vi "eval_simple_formula.vi"() -> ()   [LabVIEW 2021]
uses:
  state_def.ctl
panel:
  out "error out":errorcluster
  in  "formula":string="123"
  out "result":dbl
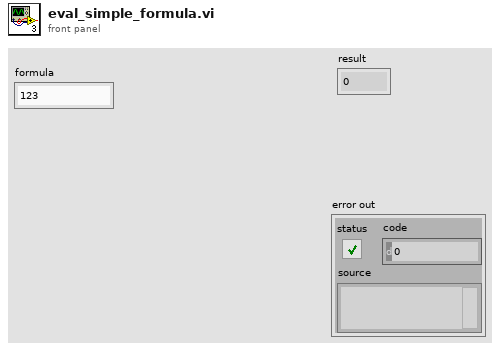
[diagram p1: front panel]
types:
  T1 = typedef "state_def.ctl" = enum16{"Init", "Construct Number", "Check Stack Priority 1", "Check Stack Priority 2", "Push", "Calculate"}
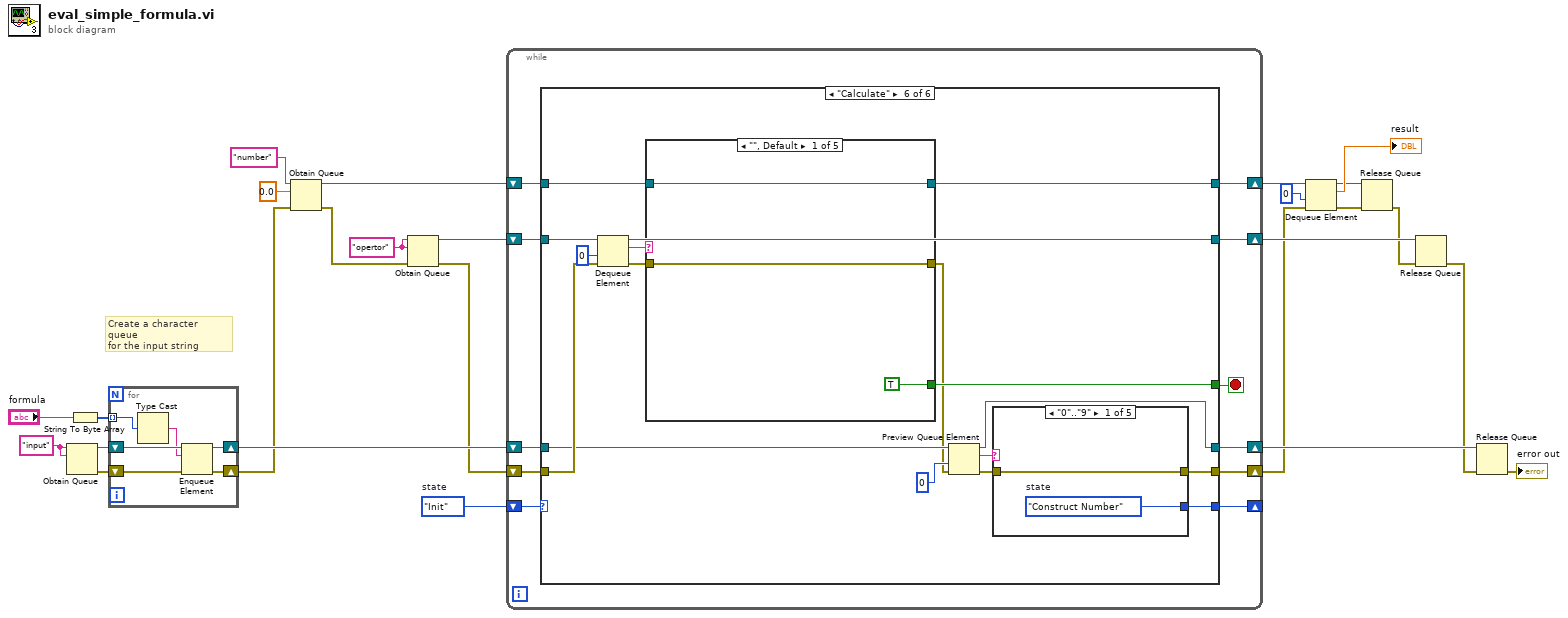
[diagram p0: block diagram]
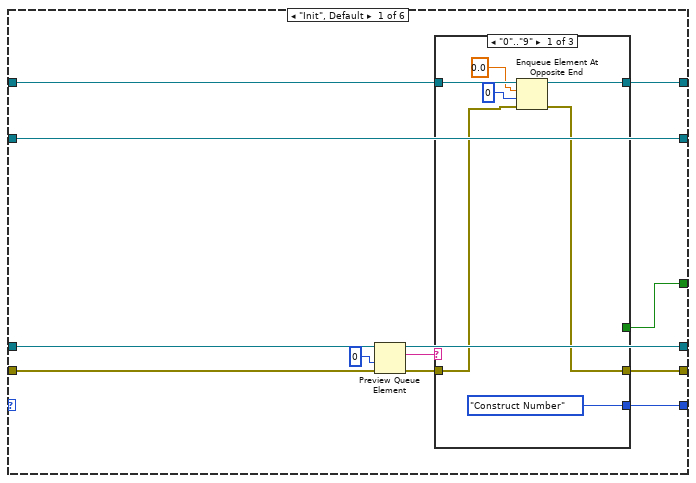
[diagram p2: hidden frame]
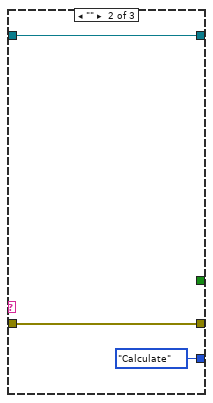
[diagram p3: hidden frame]
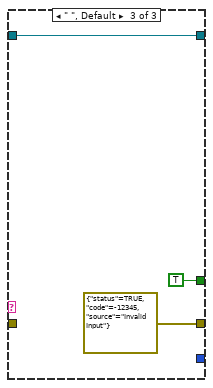
[diagram p4: hidden frame]
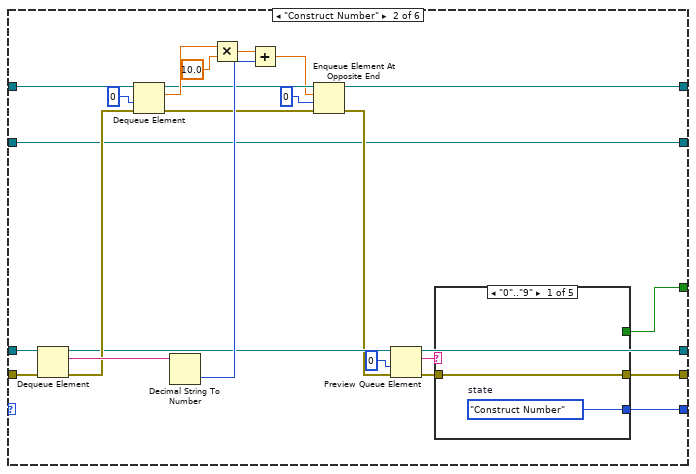
[diagram p5: hidden frame]
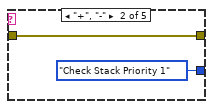
[diagram p6: hidden frame]
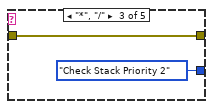
[diagram p7: hidden frame]
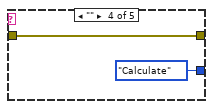
[diagram p8: hidden frame]
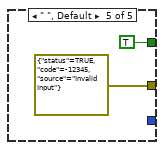
[diagram p9: hidden frame]
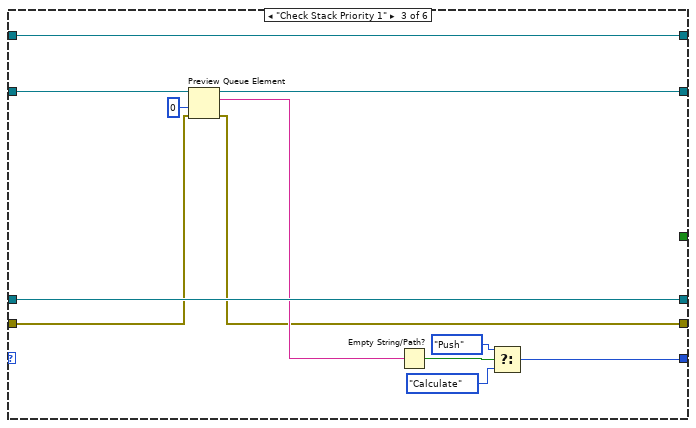
[diagram p10: hidden frame]
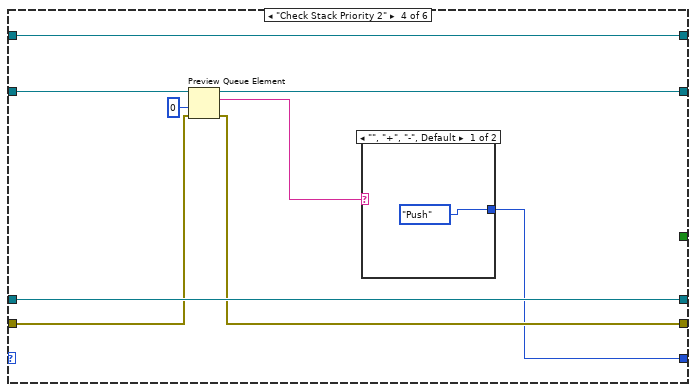
[diagram p11: hidden frame]
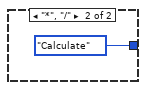
[diagram p12: hidden frame]
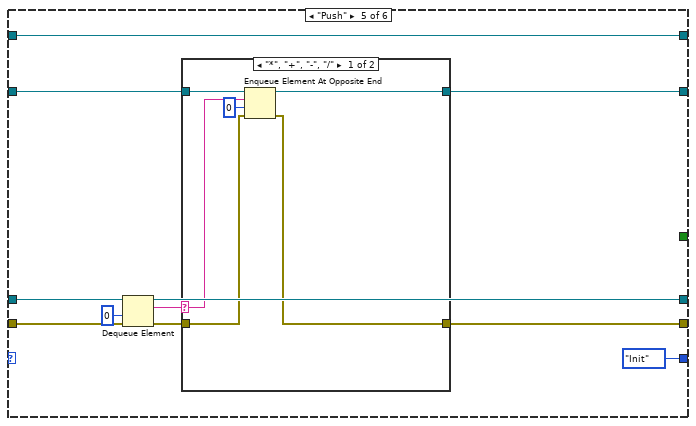
[diagram p13: hidden frame]
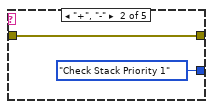
[diagram p15: hidden frame]
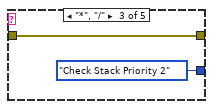
[diagram p16: hidden frame]
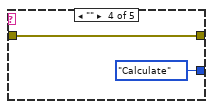
[diagram p17: hidden frame]
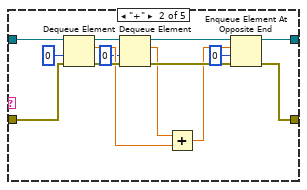
[diagram p19: hidden frame]
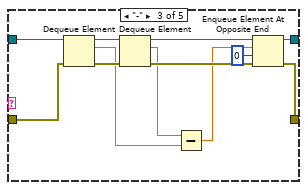
[diagram p20: hidden frame]
diagram:
  w18 = "input" ("name (unnamed)")
  w21 = "opertor" ("name (unnamed)")
  w2 = state_def."Init"  # state
  # "Create a character queue \nfor the input string"
  n1 = Obtain Queue(name (unnamed)=w18, element data type=w18) -> (queue out=w17:refnum<queue>, error out=w14:errorcluster)  [unwired: 3 in, 1 out]
  n2 = String To Byte Array(string="formula") -> (unsigned byte array=w25:u8[])
  n3 = for {
    tunnel: w25 -> [w32] mode=indexing
    shift-right: [w29] -> w16
    shift-left: w17 -> [w31]
    shift-right: [w27] -> w13
    shift-left: w14 -> [w28]
    n4 = Type Cast(x=w32) -> (*(type *) &x=w30:string)  [unwired: 1 in]
    n5 = Enqueue Element(queue=w31, element=w30, error in (no error)=w28) -> (queue out=w29:refnum<queue>, error out=w27:errorcluster)  [unwired: 1 in, 1 out]
  }
  n6 = Obtain Queue(name (unnamed)="number", element data type=0.0 ("current number"), error in (no error)=w13) -> (queue out=w22:refnum<queue>, error out=w12:errorcluster)  [unwired: 2 in, 1 out]
  n7 = Obtain Queue(name (unnamed)=w21, element data type=w21, error in (no error)=w12) -> (queue out=w20:refnum<queue>, error out=w11:errorcluster)  [unwired: 2 in, 1 out]
  n8 = while {
    shift-right: [w42] -> w8
    shift-left: w22 -> [w43]
    shift-right: [w40] -> w19
    shift-left: w20 -> [w39]
    shift-right: [w35] -> _
    shift-left: w2 -> [w33]
    shift-right: [w34] -> w15
    shift-left: w16 -> [w38]
    shift-right: [w37] -> w5
    shift-left: w11 -> [w41]
    stop <- w36 stop-if-true
    n9 = case shown="\"Calculate\"" w33 {
      tunnel: w43 -> [w55 w91 w115 w124 w137 w162]
      tunnel: [w54 w82 w115 w124 w137 w160] -> w42
      tunnel: w41 -> [w49 w81 w106 w119 w135 w157]
      tunnel: [w45 w69 w111 w120 w131 w158] -> w40
      tunnel: w39 -> [w45 w69 w113 w122 w132 w161]
      tunnel: [w53 w74 w105 w118 w130 w147] -> w37
      tunnel: [w44 w76 w114 w123 w134 w146] -> w34
      tunnel: w38 -> [w52 w93 w114 w123 w136 w150]
      tunnel: [w50 w70 _ _ _ w155] -> w36
      tunnel: [w46 w75 w108 w116 state_def."Init" ("f") w148] -> w35
      frame "Init", Default {
        n10 = Preview Queue Element(queue=w52, timeout in ms (-1)=0, error in (no error)=w49) -> (queue out=w44:refnum<queue>, element=w47:string, error out=w48:errorcluster)  [unwired: 1 out]
        n11 = case shown="\"0\"..\"9\"" w47 {
          tunnel: w55 -> [w62 w64 w66]
          tunnel: [w60 w64 w66] -> w54
          tunnel: w48 -> [w59 w65 _]
          tunnel: [w58 w65 errorcluster {"status"=TRUE, "code"=-12345, "source"="Invalid Input"} ("error out")] -> w53
          tunnel: [_ _ TRUE] -> w50
          tunnel: [state_def."Construct Number" ("state") state_def."Calculate" ("state") _] -> w46
          frame "0".."9" {
            n12 = Enqueue Element At Opposite End(queue=w62, element=0.0, timeout in ms (-1)=0, error in (no error)=w59) -> (queue out=w60:refnum<queue>, error out=w58:errorcluster)  [unwired: 1 out]
          }
          frame "" {
          }
          frame " ", Default {
          }
        }
      }
      frame "Construct Number" {
        n13 = Dequeue Element(queue=w93, error in (no error)=w81) -> (queue out=w78:refnum<queue>, element=w86:string, error out=w80:errorcluster)  [unwired: 1 in, 1 out]
        n14 = Dequeue Element(queue=w91, timeout in ms (-1)=0, error in (no error)=w80) -> (queue out=w85:refnum<queue>, element=w89:dbl, error out=w73:errorcluster)  [unwired: 1 out]
        n15 = Decimal String To Number(string=w86) -> (number=w90:i32)  [unwired: 2 in, 1 out]
        n16 = Multiply(x=w89, y=10.0) -> (x*y=w87:dbl)
        n17 = Add(x=w87, y=w90) -> (x+y=w84:dbl)
        n18 = Enqueue Element At Opposite End(queue=w85, element=w84, timeout in ms (-1)=0, error in (no error)=w73) -> (queue out=w82:refnum<queue>, error out=w72:errorcluster)  [unwired: 1 out]
        n19 = Preview Queue Element(queue=w78, timeout in ms (-1)=0, error in (no error)=w72) -> (queue out=w76:refnum<queue>, element=w77:string, error out=w71:errorcluster)  [unwired: 1 out]
        n20 = case shown="\"0\"..\"9\"" w77 {
          tunnel: [w94 w96 w98 w101 errorcluster {"status"=TRUE, "code"=-12345, "source"="Invalid Input"} ("error out")] -> w74
          tunnel: [_ _ _ _ TRUE] -> w70
          tunnel: [w95 state_def."Check Stack Priority 1" ("state") state_def."Check Stack Priority 2" ("state") state_def."Calculate" ("state") _] -> w75
          tunnel: w71 -> [w94 w96 w98 w101 _]
          frame "0".."9" {
            w95 = state_def."Construct Number"  # state
          }
          frame "+", "-" {
          }
          frame "*", "/" {
          }
          frame "" {
          }
          frame " ", Default {
          }
        }
      }
      frame "Check Stack Priority 1" {
        n21 = Preview Queue Element(queue=w113, timeout in ms (-1)=0, error in (no error)=w106) -> (queue out=w111:refnum<queue>, element=w110:string, error out=w105:errorcluster)  [unwired: 1 out]
        n22 = Empty String/Path?(string/path=w110) -> (empty?=w109:bool)
        n23 = Select(t=state_def."Push" ("state"), s=w109, f=state_def."Calculate" ("state")) -> (s? t:f=w108:T1)
      }
      frame "Check Stack Priority 2" {
        n24 = Preview Queue Element(queue=w122, timeout in ms (-1)=0, error in (no error)=w119) -> (queue out=w120:refnum<queue>, element=w117:string, error out=w118:errorcluster)  [unwired: 1 out]
        n25 = case shown="\"\", \"+\", \"-\", Default" w117 {
          tunnel: [state_def."Push" ("state") state_def."Calculate" ("state")] -> w116
          frame "", "+", "-", Default {
          }
          frame "*", "/" {
          }
        }
      }
      frame "Push" {
        n26 = Dequeue Element(queue=w136, timeout in ms (-1)=0, error in (no error)=w135) -> (queue out=w134:refnum<queue>, element=w127:string, error out=w128:errorcluster)  [unwired: 1 out]
        n27 = case shown="\"*\", \"+\", \"-\", \"/\"" w127 {
          selector: w127 -> [w138 _]
          tunnel: w132 -> [w142 w145]
          tunnel: [w141 w145] -> w131
          tunnel: [w140 w144] -> w130
          tunnel: w128 -> [w139 w144]
          frame "*", "+", "-", "/" {
            n28 = Enqueue Element At Opposite End(queue=w142, element=w138, timeout in ms (-1)=0, error in (no error)=w139) -> (queue out=w141:refnum<queue>, error out=w140:errorcluster)  [unwired: 1 out]
          }
          frame "\u0000", Default {
          }
        }
      }
      frame "Calculate" {
        n29 = Dequeue Element(queue=w161, timeout in ms (-1)=0, error in (no error)=w157) -> (queue out=w158:refnum<queue>, element=w156:string, error out=w159:errorcluster)  [unwired: 1 out]
        n30 = case shown="\"\", Default" w156 {
          tunnel: w162 -> [w174 w188 w200 w212 w224]
          tunnel: [w174 w185 w197 w209 w221] -> w160
          tunnel: w159 -> [w173 w184 w196 w208 w220]
          tunnel: [w173 w181 w193 w205 w217] -> w149
          tunnel: [TRUE _ _ _ _] -> w155
          frame "", Default {
          }
          frame "+" {
            n31 = Dequeue Element(queue=w188, timeout in ms (-1)=0, error in (no error)=w184) -> (queue out=w187:refnum<queue>, element=w179:dbl, error out=w183:errorcluster)  [unwired: 1 out]
            n32 = Dequeue Element(queue=w187, timeout in ms (-1)=0, error in (no error)=w183) -> (queue out=w186:refnum<queue>, element=w180:dbl, error out=w182:errorcluster)  [unwired: 1 out]
            n33 = Add(x=w180, y=w179) -> (x+y=w178:dbl)
            n34 = Enqueue Element At Opposite End(queue=w186, element=w178, timeout in ms (-1)=0, error in (no error)=w182) -> (queue out=w185:refnum<queue>, error out=w181:errorcluster)  [unwired: 1 out]
          }
          frame "-" {
            n35 = Dequeue Element(queue=w200, error in (no error)=w196) -> (queue out=w199:refnum<queue>, element=w191:dbl, error out=w195:errorcluster)  [unwired: 1 in, 1 out]
            n36 = Dequeue Element(queue=w199, error in (no error)=w195) -> (queue out=w198:refnum<queue>, element=w192:dbl, error out=w194:errorcluster)  [unwired: 1 in, 1 out]
            n37 = Subtract(x=w192, y=w191) -> (x-y=w190:dbl)
            n38 = Enqueue Element At Opposite End(queue=w198, element=w190, timeout in ms (-1)=0, error in (no error)=w194) -> (queue out=w197:refnum<queue>, error out=w193:errorcluster)  [unwired: 1 out]
          }
          frame "*" {
            n39 = Dequeue Element(queue=w212, error in (no error)=w208) -> (queue out=w211:refnum<queue>, element=w203:dbl, error out=w207:errorcluster)  [unwired: 1 in, 1 out]
            n40 = Dequeue Element(queue=w211, error in (no error)=w207) -> (queue out=w210:refnum<queue>, element=w204:dbl, error out=w206:errorcluster)  [unwired: 1 in, 1 out]
            n41 = Multiply(x=w204, y=w203) -> (x*y=w202:dbl)
            n42 = Enqueue Element At Opposite End(queue=w210, element=w202, timeout in ms (-1)=0, error in (no error)=w206) -> (queue out=w209:refnum<queue>, error out=w205:errorcluster)  [unwired: 1 out]
          }
          frame "/" {
            n43 = Dequeue Element(queue=w224, error in (no error)=w220) -> (queue out=w223:refnum<queue>, element=w215:dbl, error out=w219:errorcluster)  [unwired: 1 in, 1 out]
            n44 = Dequeue Element(queue=w223, error in (no error)=w219) -> (queue out=w222:refnum<queue>, element=w216:dbl, error out=w218:errorcluster)  [unwired: 1 in, 1 out]
            n45 = Divide(x=w216, y=w215) -> (x/y=w214:dbl)
            n46 = Enqueue Element At Opposite End(queue=w222, element=w214, timeout in ms (-1)=0, error in (no error)=w218) -> (queue out=w221:refnum<queue>, error out=w217:errorcluster)  [unwired: 1 out]
          }
        }
        n47 = Preview Queue Element(queue=w150, timeout in ms (-1)=0, error in (no error)=w149) -> (queue out=w146:refnum<queue>, element=w152:string, error out=w151:errorcluster)  [unwired: 1 out]
        n48 = case shown="\"0\"..\"9\"" w152 {
          tunnel: [w163 w165 w167 w170 w171] -> w147
          tunnel: [w164 state_def."Check Stack Priority 1" ("state") state_def."Check Stack Priority 2" ("state") state_def."Calculate" ("state") _] -> w148
          tunnel: w151 -> [w163 w165 w167 w170 w171]
          frame "0".."9" {
            w164 = state_def."Construct Number"  # state
          }
          frame "+", "-" {
          }
          frame "*", "/" {
          }
          frame "" {
          }
          frame " ", Default {
          }
        }
      }
    }
  }
  n49 = Dequeue Element(queue=w8, timeout in ms (-1)=0, error in (no error)=w5) -> (queue out=w3:refnum<queue>, element=→"result":dbl, error out=w4:errorcluster)  [unwired: 1 out]
  n50 = Release Queue(queue=w3, error in (no error)=w4) -> (error out=w10:errorcluster)  [unwired: 1 in, 2 out]
  n51 = Release Queue(queue=w19, error in (no error)=w10) -> (error out=w9:errorcluster)  [unwired: 1 in, 2 out]
  n52 = Release Queue(queue=w15, error in (no error)=w9) -> (error out=→"error out":errorcluster)  [unwired: 1 in, 2 out]
